vi "NI VeriStand - Open Alarm.vi"(7 "Gateway IP Address (\"\": localhost)":string, 8 "error in (no error)":errorcluster, 10 "Target Name (\"\": default target)":string, 11 "Alarm Name":string) -> (0 "error out":errorcluster, 3 "Alarm":T1)   [LabVIEW 2020, in "NI_VS Alarm ExecutionAPI.lvlib"]
doc: "Opens a reference to an alarm. You must open a reference before using any other VIs on this palette."
uses:
  <vilib>/NI VeriStand/Execution/Alarm/NI_VS Alarm ExecutionAPI.lvlib
  <vilib>/NI VeriStand/Execution/Alarm/AlarmAPI.ctl
  NationalInstruments.VeriStand.ClientAPI
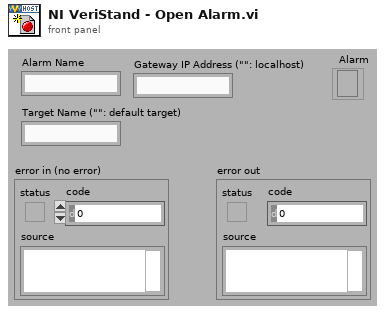
[diagram p1: front panel]
types:
  T1 = typedef "NI_VS Alarm ExecutionAPI.lvlib/AlarmAPI.ctl" = refnum<k24>
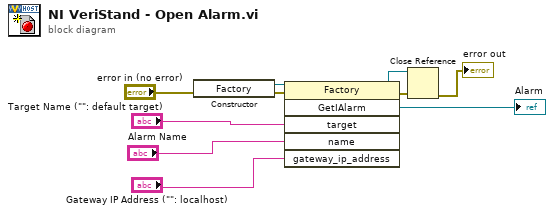
[diagram p0: block diagram]
diagram:
  n1 = constructor class="Factory"(error in="error in (no error)") -> (reference out=w8:refnum<k24>, error out=w7:errorcluster)  [unwired: 2 in, 1 out]
  n2 = invoke class="Factory" method="GetIAlarm"(reference=w8, error in=w7, "target"="Target Name (\"\": default target)", "name"="Alarm Name", "gateway_ip_address"="Gateway IP Address (\"\": localhost)") -> (reference out=w4:refnum<k24>, error out=w6:errorcluster, "GetIAlarm"=→"Alarm":refnum<k24>)  [unwired: 1 in, 3 out]
  n3 = Close Reference(reference=w4, error in (no error)=w6) -> (error out=→"error out":errorcluster)
